vi "Read ADC.vi"(8 "error in (no error)":errorcluster, 10 "ADC canal":dbl, 11 "Simulado in":refnum<class "Simulado.lvclass">) -> (0 "error out":errorcluster, 3 "Simulado out":refnum<class "Simulado.lvclass">)   [LabVIEW 2020, in "Simulado.lvclass"]
doc: "Método heredado del padre con un override"
uses:
  Simulado.lvclass
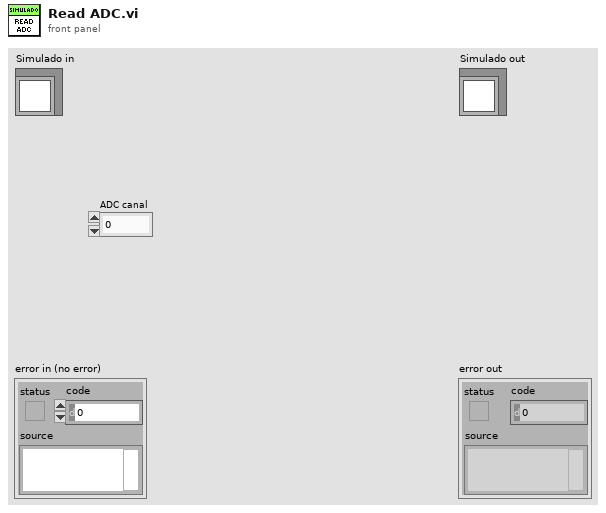
[diagram p1: front panel]
types:
  T1 = typedef "Serial device.lvclass/Brand combobox.ctl" = string
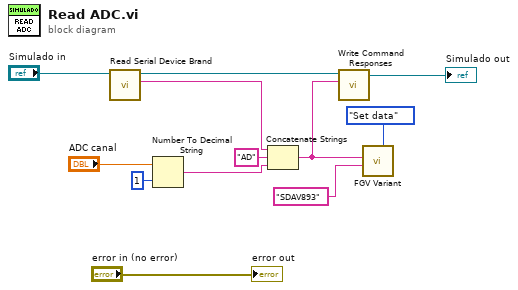
[diagram p0: block diagram]
diagram:
  n1 = call-dynamic "Read Serial Device Brand.vi"("Serial device in"="Simulado in") -> ("Serial Device Brand"=w4:T1, "Serial device out"=w8:refnum<class "Simulado.lvclass">)  [unwired: 8 in, 1 out]
  n2 = Number To Decimal String(number="ADC canal", width (-)=i16 1) -> (decimal integer string=w3:string)
  n3 = Concatenate Strings(w4, "AD" ("string"), w3) -> (w1:string)
  n4 = call-dynamic "Write Command Responses.vi"("Command Responses"=w1, "Simulado in"=w8) -> ("Simulado out"=→"Simulado out":refnum<class "Simulado.lvclass">)  [unwired: 8 in, 1 out]
  n5 = call "FGV Variant.vi"("Response to save"="SDAV893", "Command"=w1, "Functions"=enum16{"Reset data", "Set data", "Get data"}."Set data") -> ()  [unwired: 7 in, 2 out]
  "error out" <- "error in (no error)"
